vi "To Serial Form.vi"(6 "Serial Version":T1, 10 "Serializer in":refnum<class "Serializer.lvclass">, 11 "BrowerLeaf in":refnum<class "BrowerLeaf.lvclass">) -> (0 "error out":errorcluster, 2 "Serializer out":refnum<class "Serializer.lvclass">, 3 "BrowerLeaf out":refnum<class "BrowerLeaf.lvclass">)   [LabVIEW 2015, in "BrowerLeaf.lvclass"]
uses:
  BrowerLeaf.lvclass
  <vilib>/NI/AQ Character Lineator/Serializer/Serializer.lvclass
  <vilib>/NI/AQ Character Lineator/Serialization Common/Serial Version.ctl
  BrowerComponent/BrowerComponent.lvclass
  <vilib>/NI/AQ Character Lineator/Serialization Common/Serialization Common.lvlib
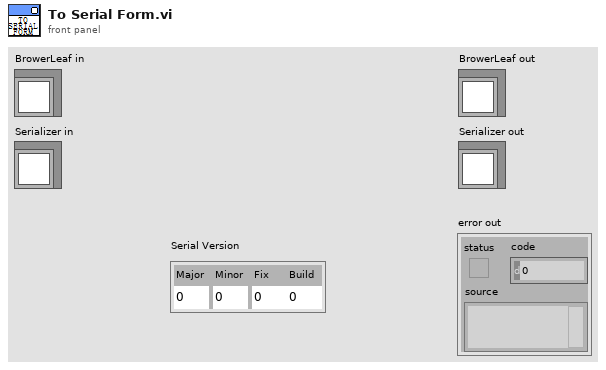
[diagram p1: front panel]
types:
  T1 = typedef "Serialization Common.lvlib/Serial Version.ctl" = cluster{"Major":u16, "Minor":u16, "Fix":u16, "Build":u16}
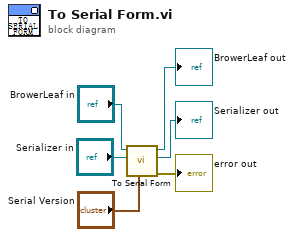
[diagram p0: block diagram]
diagram:
  n1 = call-parent "To Serial Form.vi"("Serial Version"="Serial Version", "Serializer in"="Serializer in", "BrowerComponent in"="BrowerLeaf in") -> ("error out"=→"error out":errorcluster, "Serializer out"=→"Serializer out":refnum<class "Serializer.lvclass">, "BrowerComponent out"=→"BrowerLeaf out":refnum<class "BrowerLeaf.lvclass">)  [unwired: 6 in]
